vi "Page_Source_Settings_Update_Display.vi"(6 "AB_Build in":refnum<class "AB_Build.lvclass">, 8 "error in (no error)":errorcluster, 9 "ctlReferences":T3, 10 "supportedFunctions":T2, 11 "AB_Source_VI in":refnum<class "AB_Source_VI.lvclass">) -> (0 "error out":errorcluster, 2 "parentApplies":T1, 3 "AB_Source_VI out":refnum<class "AB_Source_VI.lvclass">)   [LabVIEW 2020, in "AB_Source_VI.lvclass"]
uses:
  <vilib>/AppBuilder/AB_Classes/Source/VI/AB_Source_VI.lvclass
  e:/builds/penguin/labview/branches/2020/dev/dist/vi.lib/AppBuilder/AB_Classes/Source/AB_Source.lvclass
  <resource>/Framework/Providers/Builds/AppBuilder/AB_UI_Page_Source_Settings_References.ctl
  <resource>/Framework/Providers/Builds/AppBuilder/AB_UI_Page_Source_Settings_supportedFunctions.ctl
  <vilib>/AppBuilder/AB_Parent_Applies.ctl
  <vilib>/AppBuilder/AB_Classes/Build/AB_Build.lvclass
  <vilib>/AppBuilder/AB_Source_Inclusion.ctl
  <vilib>/AppBuilder/AB_Classes/Source/VI/AB_Source_VI.lvclass/AB_Source_VI.ctl
  <vilib>/AppBuilder/AB_Classes/Source/AB_Source.lvclass
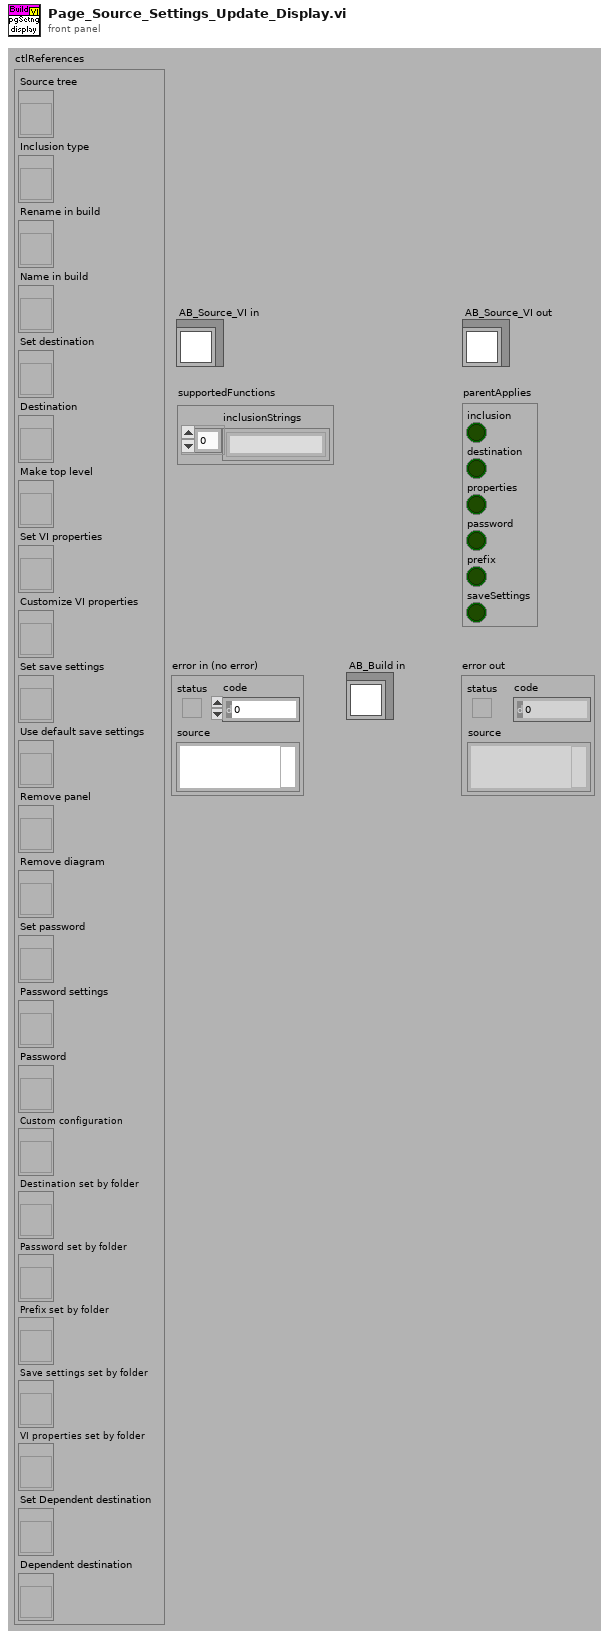
[diagram p1: front panel]
types:
  T1 = typedef "AB_Parent_Applies.ctl" = cluster{"inclusion":bool, "destination":bool, "properties":bool, "password":bool, "prefix":bool, "saveSettings":bool}
  T2 = typedef "AB_UI_Page_Source_Settings_supportedFunctions.ctl" = cluster{"inclusionStrings":string[]}
  T3 = typedef "AB_UI_Page_Source_Settings_References.ctl" = cluster{"Source tree":refnum<vi>, "Inclusion type":refnum<vi>, "Rename in build":refnum<vi>, "Name in build":refnum<vi>, "Set destination":refnum<vi>, "Destination":refnum<vi>, "Make top level":refnum<vi>, "Set VI properties":refnum<vi>, "Customize VI properties":refnum<vi>, "Set save settings":refnum<vi>, "Use default save settings":refnum<vi>, "Remove panel":refnum<vi>, "Remove diagram":refnum<vi>, "Set password":refnum<vi>, "Password settings":refnum<vi>, "Password":refnum<vi>, "Custom configuration":refnum<vi>, "Destination set by folder":refnum<vi>, "Password set by folder":refnum<vi>, "Prefix set by folder":refnum<vi>, "Save settings set by folder":refnum<vi>, "VI properties set by folder":refnum<vi>, "Set Dependent destination":refnum<vi>, "Dependent destination":refnum<vi>}
  T4 = typedef "AB_Source_Inclusion.ctl" = enum16{"IncludeIfReferenced", "Include", "Exclude", "TopLevel"}
  T5 = typedef "AB_Source.ctl" = cluster{"path":path, "itemID":string, "parentIndex":i32, "sourceInclusion":T4, "destinationIndex":i32, "properties":T6[], "newName":string, "lvfile":bool, "valid":bool, "eng_inBuild":bool, "eng_isNonVILink":bool, "Amalgamation":bool, "Amalgamation Piece":bool, "eng_delimitedName":string, "preventRename":bool}
  T6 = typedef "AB_Source_Properties.ctl" = cluster{"sourcePropertyType":T7, "value":variant}
  T7 = typedef "AB_Source_Property_Type.ctl" = enum16{"Remove block diagram", "Remove front panel", "Password", "Window has title bar", "Show menu bar", "Show vertical scroll bar", "Show horizontal scroll bar", "Show toolbar", "Show Abort button", "Show fp when called", "Window behavior", "Allow user to close window", "Window run-time position", "Run when opened", "Allow debugging", "Auto error handling", "Generate guard code", "Use stack variables", "Expression folding", "Integer only", "Inline subVI"}
  T8 = enum32{"No password change", "Remove password", "Apply new password"}
  T9 = typedef "AB_Build.ctl" = cluster{"buildSpecName":string, "buildSpecDescription":string, "destinations":refnum<class "AB_Destination.lvclass">[], "exclusionOption":T10, "defaultLanguage":string, "supportedLanguages":string[], "excludedDirectories":path[], "buildContext":refnum<vi>, "buildObject":T11, "preview":bool, "programatic":bool, "progressBarEvents":T12, "userLog_Path":path, "preActionID":string, "preAction_Path":path, "postActionID":string, "postAction_Path":path, "eng_checkForBrokenVIs?":bool, "eng_verboseLinkerErrors?":bool, "localDest_Path":path, "targetDest_Path":path, "removeVIObject":u16, "cache":refnum<class "PreviewCache.lvclass">, "use cache":bool, "previewCache_ID":string, "buildCache_ID":string, "eng_TempLocalDest_Path":path, "eng_collectDependencies?":bool, "versionInfo":cluster{"buildVersion":cluster{"major":u16, "minor":u16, "patch":u16, "build":u16}, "autoIncrement":bool}, "eng_enableVIChecksums":bool}
  T10 = typedef "AB_Exclusion_Option.ctl" = cluster{"typedefs":bool, "polymorphicVIs":bool, "unusedLibraryItems":bool, "modifyLibraryFile":bool, "edit-timeDependencies":bool, "inlineVIs":bool, "dependent PPLs":bool, "dependent DLLs":bool}
  T11 = typedef "ItemRef.ctl" = u64
  T12 = typedef "provcom_ProgressBar_Events.ctl" = cluster{"newJob":refnum<user-event>, "newItem":refnum<user-event>, "errorMsg":T13, "cancel":refnum<user-event>}
  T13 = typedef "mxLvBuildError.ctl" = refnum<user-event>
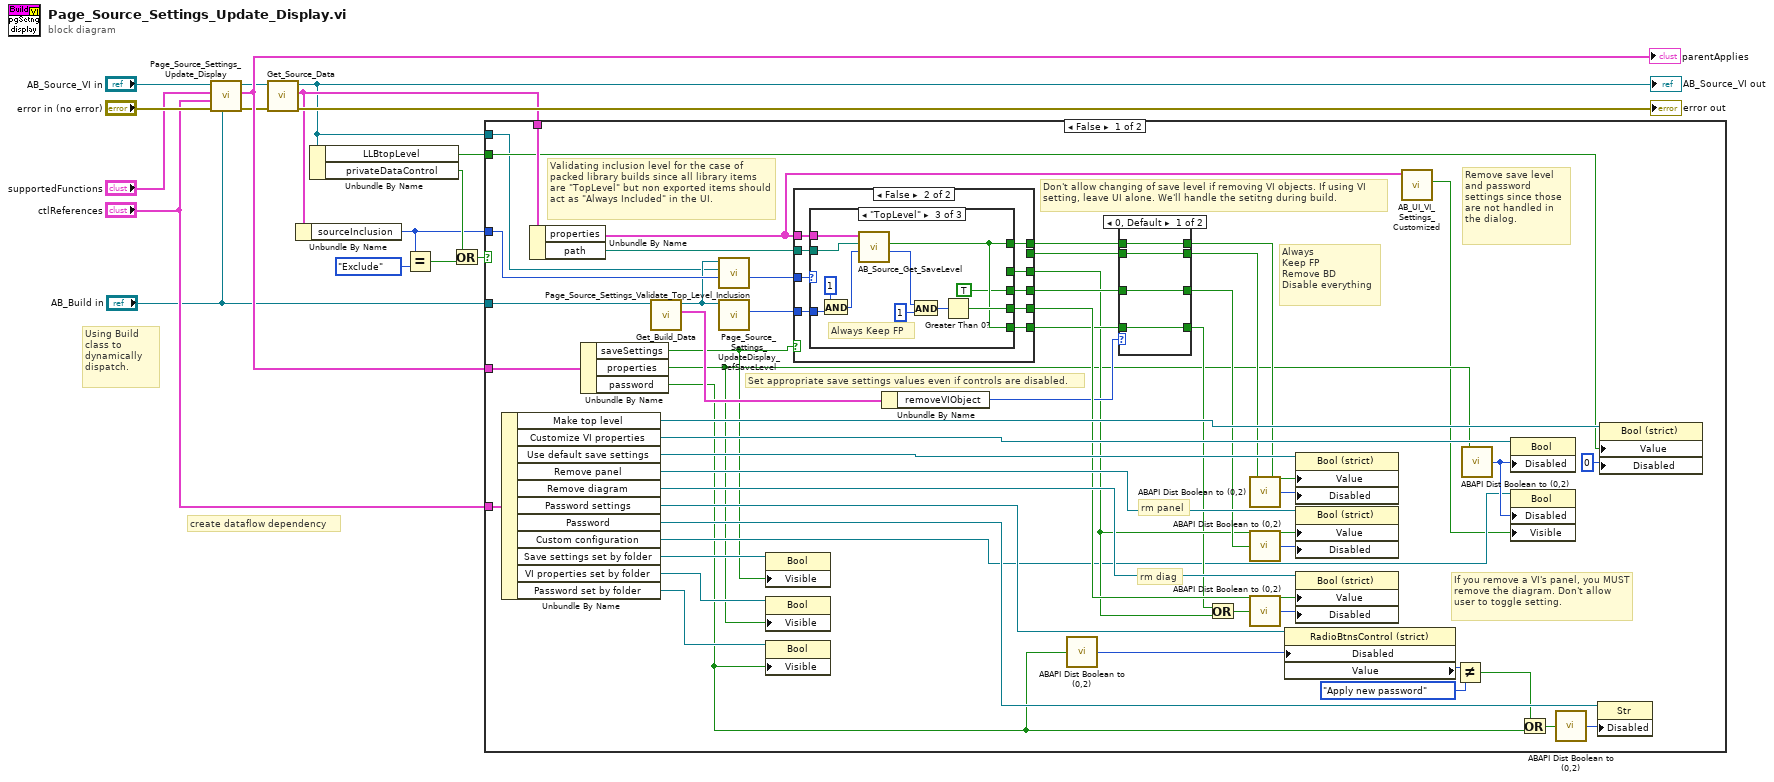
[diagram p0: block diagram]
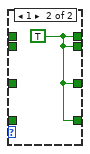
[diagram p2: hidden frame]
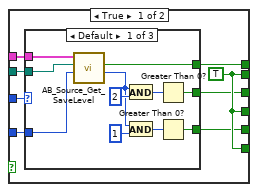
[diagram p3: hidden frame]
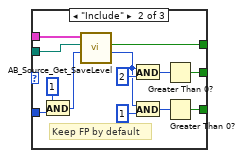
[diagram p4: hidden frame]
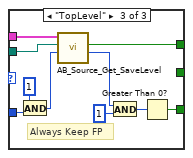
[diagram p5: hidden frame]
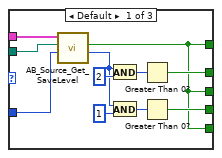
[diagram p6: hidden frame]
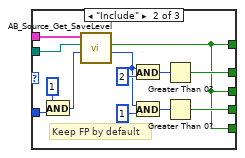
[diagram p7: hidden frame]
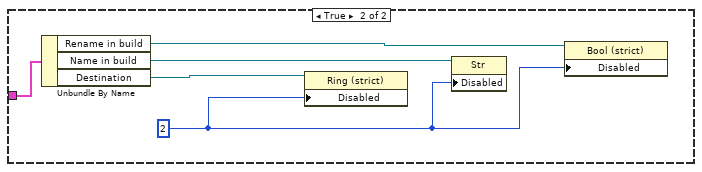
[diagram p8: hidden frame]
diagram:
  # "Using Build class to dynamically dispatch."
  # "create dataflow dependency"
  n1 = call-parent "Page_Source_Settings_Update_Display.vi"("AB_Build in"="AB_Build in", "error in (no error)"="error in (no error)", "ctlReferences"="ctlReferences", "supportedFunctions"="supportedFunctions", "AB_Source in"="AB_Source_VI in") -> ("error out"=w11:errorcluster, "parentApplies"=w14:T1, "AB_Source out"=w12:refnum<class "AB_Source_VI.lvclass">)  [unwired: 4 in]
  "parentApplies" <- w14
  n2 = call <vilib>:"Get_Source_Data.vi"("error in (no error)"=w11, "Class in"=w12) -> ("error out"=→"error out":errorcluster, "data"=w8:T5, "Class out"=w1:refnum<class "AB_Source_VI.lvclass">)  [unwired: 7 in]
  "AB_Source_VI out" <- w1
  n3 = Unbundle By Name(w8) -> ("sourceInclusion"=w2:T4)
  n4 = Unbundle By Name(w1) -> ("LLBtopLevel"=w9:bool, "privateDataControl"=w7:bool)
  n5 = Equal?(x=w2, y=AB_Source_Inclusion."Exclude") -> (x = y?=w4:bool)
  n6 = Or(x=w7, y=w4) -> (x .or. y?=w6:bool)
  n7 = case shown="False" w6 {
    tunnel: "ctlReferences" -> [w68 w164]
    tunnel: w14 -> [w57 _]
    tunnel: w8 -> [w50 _]
    tunnel: w9 -> [w48 _]
    tunnel: "AB_Build in" -> [w44 _]
    tunnel: w2 -> [w23 _]
    tunnel: w1 -> [w20 _]
    frame False {
      # "Don't allow changing of save level if removing VI objects. If using VI setting, leave UI alone. We'll handle the setitng during build."
      # "Remove save level and password settings since those are not handled in the dialog."
      # "Validating inclusion level for the case of packed library builds since all library items are \"TopLevel\" but non exported items should act as \"Always Included\" in the UI."
      # "Set appropriate save settings values even if controls are disabled."
      # "rm diag"
      # "rm panel"
      # "If you remove a VI's panel, you MUST remove the diagram. Don't allow user to toggle setting."
      # "Always\nKeep FP\nRemove BD\nDisable everything"
      n8 = Unbundle By Name(w68) -> ("Make top level"=w64:refnum<vi>, "Customize VI properties"=w67:refnum<vi>, "Use default save settings"=w56:refnum<vi>, "Remove panel"=w54:refnum<vi>, "Remove diagram"=w53:refnum<vi>, "Password settings"=w66:refnum<vi>, "Password"=w65:refnum<vi>, "Custom configuration"=w30:refnum<vi>, "Save settings set by folder"=w29:refnum<vi>, "VI properties set by folder"=w28:refnum<vi>, "Password set by folder"=w27:refnum<vi>)
      n9 = Unbundle By Name(w50) -> ("properties"=w19:T6[], "path"=w47:path)
      n10 = Unbundle By Name(w57) -> ("saveSettings"=w26:bool, "properties"=w25:bool, "password"=w24:bool)
      n11 = call <vilib>:"Get_Build_Data.vi"("Class in"=w44) -> ("data"=w43:T9, "Class out"=w21:refnum<class "AB_Build.lvclass">)  [unwired: 8 in, 1 out]
      n12 = call-dynamic "Page_Source_Settings_Validate_Top_Level_Inclusion.vi"("sourceInclusion in"=w23, "AB_Source in"=w20, "AB_Build in"=w21) -> ("sourceInclusion out"=w22:T4)  [unwired: 6 in, 2 out]
      n13 = call-dynamic "Page_Source_Settings_UpdateDisplay_DefSaveLevel.vi"("AB_Build in"=w21) -> ("defaultSaveLevel"=w45:u32)  [unwired: 8 in, 2 out]
      n14 = property class="Bool"(reference=w29, "Visible"=w26) -> ()  [unwired: 1 in, 2 out]
      n15 = property class="Bool"(reference=w28, "Visible"=w25) -> ()  [unwired: 1 in, 2 out]
      n16 = property class="Bool"(reference=w27, "Visible"=w24) -> ()  [unwired: 1 in, 2 out]
      n17 = case shown="False" w26 {
        tunnel: w22 -> [w79 w117]
        tunnel: w19 -> [w80 w124]
        tunnel: [w76 w123] -> w41
        tunnel: [w81 _] -> w40
        tunnel: [w81 w122] -> w37
        tunnel: [w81 w121] -> w36
        tunnel: w45 -> [w77 w120]
        tunnel: [w75 w119] -> w34
        tunnel: [w74 w118] -> w49
        tunnel: w47 -> [w78 w116]
        frame True {
          w81 = TRUE
          n18 = case shown="Default" w79 {
            tunnel: w80 -> [w92 w105 w115]
            tunnel: [w83 w94 w107] -> w76
            tunnel: w77 -> [w91 w101 w111]
            tunnel: [w88 w96 _] -> w75
            tunnel: [w84 w102 w112] -> w74
            tunnel: w78 -> [w82 w93 w106]
            frame Default {
              n19 = call <vilib>:"AB_Source_Get_SaveLevel.vi"("defaultSaveLevel"=w91, "VIpath"=w82, "sourceProperties in"=w92) -> ("saveLevel out"=w85:u32, "useDefault"=w83:bool)  [unwired: 5 in, 2 out]
              n20 = And(x=w85, y=u32 2) -> (x .and. y?=w89:u32)
              n21 = And(x=w85, y=u32 1) -> (x .and. y?=w87:u32)
              n22 = Greater Than 0?(x=w89) -> (x > 0?=w88:bool)
              n23 = Greater Than 0?(x=w87) -> (x > 0?=w84:bool)
            }
            frame "Include" {
              # "Keep FP by default"
              n24 = And(x=u32 1 ("defaultSaveLevel"), y=w101) -> (x .and. y?=w100:u32)
              n25 = call <vilib>:"AB_Source_Get_SaveLevel.vi"("defaultSaveLevel"=w100, "VIpath"=w93, "sourceProperties in"=w105) -> ("saveLevel out"=w95:u32, "useDefault"=w94:bool)  [unwired: 5 in, 2 out]
              n26 = And(x=w95, y=u32 2) -> (x .and. y?=w97:u32)
              n27 = And(x=w95, y=u32 1) -> (x .and. y?=w104:u32)
              n28 = Greater Than 0?(x=w97) -> (x > 0?=w96:bool)
              n29 = Greater Than 0?(x=w104) -> (x > 0?=w102:bool)
            }
            frame "TopLevel" {
              # "Always Keep FP"
              n30 = And(x=u32 1 ("defaultSaveLevel"), y=w111) -> (x .and. y?=w110:u32)
              n31 = call <vilib>:"AB_Source_Get_SaveLevel.vi"("defaultSaveLevel"=w110, "VIpath"=w106, "sourceProperties in"=w115) -> ("saveLevel out"=w108:u32, "useDefault"=w107:bool)  [unwired: 5 in, 2 out]
              n32 = And(x=w108, y=u32 1) -> (x .and. y?=w114:u32)
              n33 = Greater Than 0?(x=w114) -> (x > 0?=w112:bool)
            }
          }
        }
        frame False {
          n34 = case shown="\"TopLevel\"" w117 {
            tunnel: w124 -> [w135 w148 w159]
            tunnel: [w126 w137 w151] -> w123
            tunnel: [w126 w137 TRUE ("useDefault")] -> w122
            tunnel: [w126 w137 w151] -> w121
            tunnel: w120 -> [w134 w144 w155]
            tunnel: [w131 w139 _] -> w119
            tunnel: [w127 w145 w156] -> w118
            tunnel: w116 -> [w125 w136 w149]
            frame Default {
              n35 = call <vilib>:"AB_Source_Get_SaveLevel.vi"("defaultSaveLevel"=w134, "VIpath"=w125, "sourceProperties in"=w135) -> ("saveLevel out"=w128:u32, "useDefault"=w126:bool)  [unwired: 5 in, 2 out]
              n36 = And(x=w128, y=u32 2) -> (x .and. y?=w132:u32)
              n37 = And(x=w128, y=u32 1) -> (x .and. y?=w130:u32)
              n38 = Greater Than 0?(x=w132) -> (x > 0?=w131:bool)
              n39 = Greater Than 0?(x=w130) -> (x > 0?=w127:bool)
            }
            frame "Include" {
              # "Keep FP by default"
              n40 = And(x=u32 1 ("defaultSaveLevel"), y=w144) -> (x .and. y?=w143:u32)
              n41 = call <vilib>:"AB_Source_Get_SaveLevel.vi"("defaultSaveLevel"=w143, "VIpath"=w136, "sourceProperties in"=w148) -> ("saveLevel out"=w138:u32, "useDefault"=w137:bool)  [unwired: 5 in, 2 out]
              n42 = And(x=w138, y=u32 2) -> (x .and. y?=w140:u32)
              n43 = And(x=w138, y=u32 1) -> (x .and. y?=w147:u32)
              n44 = Greater Than 0?(x=w140) -> (x > 0?=w139:bool)
              n45 = Greater Than 0?(x=w147) -> (x > 0?=w145:bool)
            }
            frame "TopLevel" {
              # "Always Keep FP"
              n46 = And(x=u32 1 ("defaultSaveLevel"), y=w155) -> (x .and. y?=w154:u32)
              n47 = call <vilib>:"AB_Source_Get_SaveLevel.vi"("defaultSaveLevel"=w154, "VIpath"=w149, "sourceProperties in"=w159) -> ("saveLevel out"=w152:u32, "useDefault"=w151:bool)  [unwired: 5 in, 2 out]
              n48 = And(x=w152, y=u32 1) -> (x .and. y?=w158:u32)
              n49 = Greater Than 0?(x=w158) -> (x > 0?=w156:bool)
            }
          }
        }
      }
      n50 = Unbundle By Name(w43) -> ("removeVIObject"=w42:u16)
      n51 = call <vilib>:"ABAPI Dist Boolean to (0,2).vi"("Boolean"=w24) -> ("0, 2"=w58:u8)  [unwired: 4 in]
      n52 = case shown="0, Default" w42 {
        tunnel: w41 -> [w72 _]
        tunnel: [w72 w73] -> w39
        tunnel: w40 -> [w71 _]
        tunnel: [w71 w73] -> w38
        tunnel: w37 -> [w70 _]
        tunnel: w36 -> [w69 _]
        tunnel: [w70 w73] -> w35
        tunnel: [w69 w73] -> w33
        frame 0, Default {
        }
        frame 1 {
          w73 = TRUE ("useDefault")
        }
      }
      n53 = Or(x=w33, y=w34) -> (x .or. y?=w32:bool)
      n54 = call <vilib>:"ABAPI Dist Boolean to (0,2).vi"("Boolean"=w38) -> ("0, 2"=w55:u8)  [unwired: 4 in]
      n55 = call <vilib>:"ABAPI Dist Boolean to (0,2).vi"("Boolean"=w35) -> ("0, 2"=w52:u8)  [unwired: 4 in]
      n56 = call <vilib>:"ABAPI Dist Boolean to (0,2).vi"("Boolean"=w32) -> ("0, 2"=w51:u8)  [unwired: 4 in]
      n57 = property class="RadioBtnsControl (strict)"(reference=w66, "Disabled"=w58) -> ("Value"=w63:T8)  [unwired: 1 in, 2 out]
      n58 = property class="Bool (strict)"(reference=w56, "Value"=w39, "Disabled"=w55) -> ()  [unwired: 1 in, 2 out]
      n59 = property class="Bool (strict)"(reference=w54, "Value"=w34, "Disabled"=w52) -> ()  [unwired: 1 in, 2 out]
      n60 = property class="Bool (strict)"(reference=w53, "Value"=w49, "Disabled"=w51) -> ()  [unwired: 1 in, 2 out]
      n61 = call <resource>:"AB_UI_VI_Settings_Customized.vi"("sourceProperties in"=w19) -> ("customized"=w18:bool)  [unwired: 9 in, 1 out]
      n62 = Not Equal?(x=w63, y=T8."Apply new password") -> (x != y?=w61:bool)
      n63 = call <vilib>:"ABAPI Dist Boolean to (0,2).vi"("Boolean"=w25) -> ("0, 2"=w31:u8)  [unwired: 4 in]
      n64 = property class="Bool"(reference=w67, "Disabled"=w31) -> ()  [unwired: 1 in, 2 out]
      n65 = property class="Bool"(reference=w30, "Disabled"=w31, "Visible"=w18) -> ()  [unwired: 1 in, 2 out]
      n66 = Or(x=w61, y=w24) -> (x .or. y?=w60:bool)
      n67 = call <vilib>:"ABAPI Dist Boolean to (0,2).vi"("Boolean"=w60) -> ("0, 2"=w59:u8)  [unwired: 4 in]
      n68 = property class="Str"(reference=w65, "Disabled"=w59) -> ()  [unwired: 1 in, 2 out]
      n69 = property class="Bool (strict)"(reference=w64, "Value"=w48, "Disabled"=u8 0) -> ()  [unwired: 1 in, 2 out]
    }
    frame True {
      w160 = u8 2 ("Disabled")
      n70 = Unbundle By Name(w164) -> ("Rename in build"=w161:refnum<vi>, "Name in build"=w162:refnum<vi>, "Destination"=w163:refnum<vi>)
      n71 = property class="Ring (strict)"(reference=w163, "Disabled"=w160) -> ()  [unwired: 1 in, 2 out]
      n72 = property class="Str"(reference=w162, "Disabled"=w160) -> ()  [unwired: 1 in, 2 out]
      n73 = property class="Bool (strict)"(reference=w161, "Disabled"=w160) -> ()  [unwired: 1 in, 2 out]
    }
  }
